vi "Write.Data.Commit.vi"(8 "error in (no error)":errorcluster, 11 "Ref":T1) -> (0 "error out":errorcluster)   [LabVIEW 2015, in "Data Access Engine.lvlib" / "Data Access Engine.lvclass"]
uses:
  Data Access Engine.lvclass
  Types/Write.DVR.ctl
  Access Type Classes/Write/Write.lvclass
  Access Type Classes/Write/Write.lvclass/Write.ctl
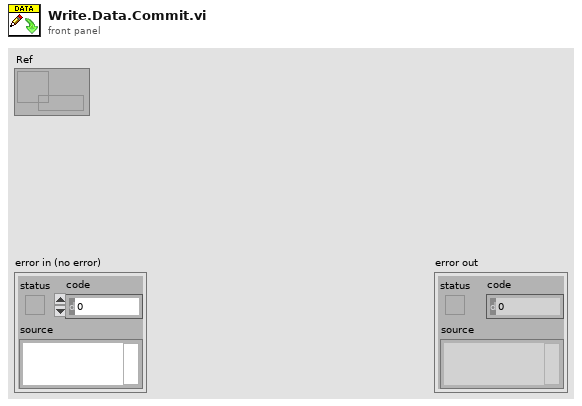
[diagram p1: front panel]
types:
  T1 = typedef "Data Access Engine.lvlib/Data Access Engine.lvclass/Write.DVR.ctl" = refnum<data-value>
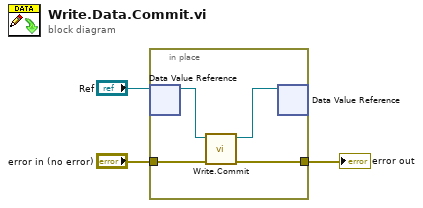
[diagram p0: block diagram]
diagram:
  n1 = in-place {
    in-place-border: "error in (no error)" -> [w7]
    in-place-border: [w6] -> w2
    n2 = in-place-dvr #1("Ref") -> (w5:refnum<class "Write.lvclass">)  [unwired: 1 out]
    n3 = call "Write.Commit.vi"("error in (no error)"=w7, "Write in"=w5) -> ("error out"=w6:errorcluster, "Write out"=w4:refnum<class "Write.lvclass">)  [unwired: 8 in]
    n4 = in-place-dvr #1(w4) -> ()  [unwired: 2 out]
  }
  "error out" <- w2
